vi "Rotation3d_Create_Quaternion.vi"(11 "Quaternion":T2={"R"=1.0, "V"=[0.0, 0.0, 0.0]}) -> (3 "Rotation3d":T1={"Q_quaternion"={"R"=1.0, "V"=[0.0, 0.0, 0.0]}})   [LabVIEW 2019, in "Trajectory_Library.lvlib"]
doc: "Constructs a Rotation3d from a quaternion.\n\nParmeters:\n -Quaternion - The quaternion to convert to Rotation3d.\n\nReturns\n - Rotation3d -- Rotation3d data structure"
uses:
  Trajectory_Library.lvlib
  TypeDef/QUATERNION.ctl
  TypeDef/ROTATION3D.ctl
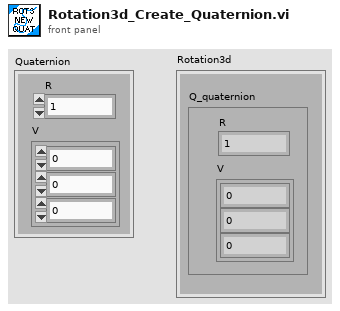
[diagram p1: front panel]
types:
  T1 = typedef "Trajectory_Library.lvlib/ROTATION3D.ctl" = cluster{"Q_quaternion":T2}
  T2 = typedef "Trajectory_Library.lvlib/QUATERNION.ctl" = cluster{"R":dbl, "V":dbl[]}
  T3 = typedef "WPILib_Math.lvlib/QUATERNION.ctl" = cluster{"R":dbl, "V":dbl[]}
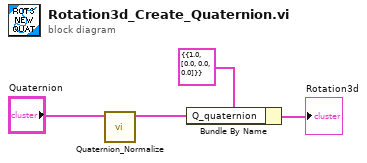
[diagram p0: block diagram]
diagram:
  n1 = call "Quaternion_Normalize.vi"("Quaternion"="Quaternion") -> ("Normalize"=w2:T3)  [unwired: 10 in]
  n2 = Bundle By Name(cluster=T1 {"Q_quaternion"={"R"=1.0, "V"=[0.0, 0.0, 0.0]}} ("ROTATION3D"), "Q_quaternion"=w2) -> (→"Rotation3d":T1)
